vi "Begin.vi"(8 "error in":errorcluster) -> (0 "error out":errorcluster)   [LabVIEW 2020]
doc: "Called before other user functions, this VI can be used to open I/O refnums, load in file data, and do general program initialization. Notice that the <B>error out</B> terminal is simply used for data flow. Wiring it to other structures or subVIs ensures that this VI runs first."
uses:
  <vilib>/Rock Robotics/WPI/DriverStation/WPI_DriverStationRobotMode2.ctl
  <vilib>/Rock Robotics/WPI/Joystick/WPI_JoystickDeviceEnum.ctl
  Robot Global Data.vi
  <vilib>/Rock Robotics/Network Tables/NT Write String Array.vi
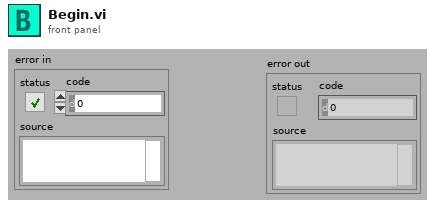
[diagram p1: front panel]
types:
  T1 = typedef "WPI_JoystickDeviceEnum.ctl" = enum16{"USB 0", "USB 1", "USB 2", "USB 3", "USB 4", "USB 5"}
  T2 = typedef "WPI_DriverStationRobotMode2.ctl" = enum16{"Autonomous Disabled", "Autonomous Enabled", "Teleop Disabled", "Teleop Enabled", "Disconnected", "Finish", "Test Disabled", "Test Enabled", "Emergency Stopped"}
  T3 = typedef "WPI_JoystickDevRef.ctl" = cluster{"Device":T1}
  T4 = typedef "numlock.ctl" = cluster{"tdms file out":refnum<k34>, "Default log level (info)":enum16{"trace", "debug", "info", "warn", "error"}}
  T5 = typedef "CTRE_PigeonIMU_DeviceRef.ctl" = cluster{"DeviceStatus":errorcluster, "Device Number":u8, "Type":T6, "Device ID":u32, "Handle":u64, "UsageFrame":u32, "Library Path":path}
  T6 = typedef "CTRE_PigeonIMU_ConnectionType.ctl" = u32
  T7 = typedef "ADIS16470 Device Reference.ctl" = cluster{"DevStatus":errorcluster, "Hardware Config":T8, "Calibration Complete":refnum<notifier>, "Status Reference":refnum<data-value>, "Position Reference":refnum<data-value>, "Velocity Reference":refnum<data-value>, "Sychronous Process VI":T12, "Cmd FIFO":refnum<k33>, "Source":T13, "Data FIFO":refnum<k33>, "Calibration Time (ms)":u32}
  T8 = typedef "ADIS16470 Hardware Configuration.ctl" = cluster{"SPI Clock Rate (Hz)":dbl, "IMU SPI Mode (3)":T9, "IMU Reset Pin":T10, "IMU SPI Bus":T11, "IMU Data Ready Pin":T10, "Stall Config":cluster{"Pow2BytesPerRead":u8, "StallTicks":u16, "CsToSclkTicks":u8}}
  T9 = typedef "WPI_SPIMode.ctl" = enum16{"Mode 0 (Clk Idle Low,Sample on Leading)", "Mode 1 (Clk Idle Low,Sample on Trailing)", "Mode 2 (Clk Idle High,Sample on Leading)", "Mode 3 (Clk Idle High,Sample on Trailing)"}
  T10 = typedef "FPGA_DIOChannel.ctl" = enum8{"DIO 0", "DIO 1", "DIO 2", "DIO 3", "DIO 4", "DIO 5", "DIO 6", "DIO 7", "DIO 8", "DIO 9", "DIO MXP 0", "DIO MXP 1", "DIO MXP 2", "DIO MXP 3", "DIO MXP 4", "DIO MXP 5", "DIO MXP 6", "DIO MXP 7", "DIO MXP 8", "DIO MXP 9", "DIO MXP 10", "DIO MXP 11", "DIO MXP 12", "DIO MXP 13", "DIO MXP 14", "DIO MXP 15", "SPI Port CS1", "SPI Port CS2", "SPI Port CS3", "SPI Port MISO", "SPI Port MOSI", "Invalid"}
  T11 = typedef "spi_bus.ctl" = enum16{"SPI On-Board, CS0", "SPI On-Board, CS1", "SPI On-Board, CS2", "SPI On-Board, CS3", "SPI MXP", "Invalid"}
  T12 = typedef "ADIS16470 Process.ctl" = refnum<vi>
  T13 = typedef "FPGA_CounterEncoderSourceConvertionLVSourceType.ctl" = cluster{"DevStatus":errorcluster, "AnalogTriggerMode?":bool, "DigitalMode":cluster{"DIO Channel":T14}, "AnalogTriggerMode":cluster{"AnalogTriggerIndex":T15, "OutputType":T16}}
  T14 = typedef "FPGA_DIODigitalSourceChannel.ctl" = enum8{"DIO 0", "DIO 1", "DIO 2", "DIO 3", "DIO 4", "DIO 5", "DIO 6", "DIO 7", "DIO 8", "DIO 9", "DIO MXP 0", "DIO MXP 1", "DIO MXP 2", "DIO MXP 3", "DIO MXP 4", "DIO MXP 5", "DIO MXP 6", "DIO MXP 7", "DIO MXP 8", "DIO MXP 9", "DIO MXP 10", "DIO MXP 11", "DIO MXP 12", "DIO MXP 13", "DIO MXP 14", "DIO MXP 15", "SPI Port CS1", "SPI Port CS2", "SPI Port CS3", "SPI Port MISO", "SPI Port MOSI", "Disabled"}
  T15 = typedef "FPGA_AnalogTriggerIndex.ctl" = enum8{"Trig 0", "Trig 1", "Trig 2", "Trig 3", "Trig 4", "Trig 5", "Trig 6", "Trig 7", "Invalid"}
  T16 = typedef "FPGA_AnalogTriggerOutType.ctl" = enum16{"InWindow", "TriggerState", "Rising", "Falling"}
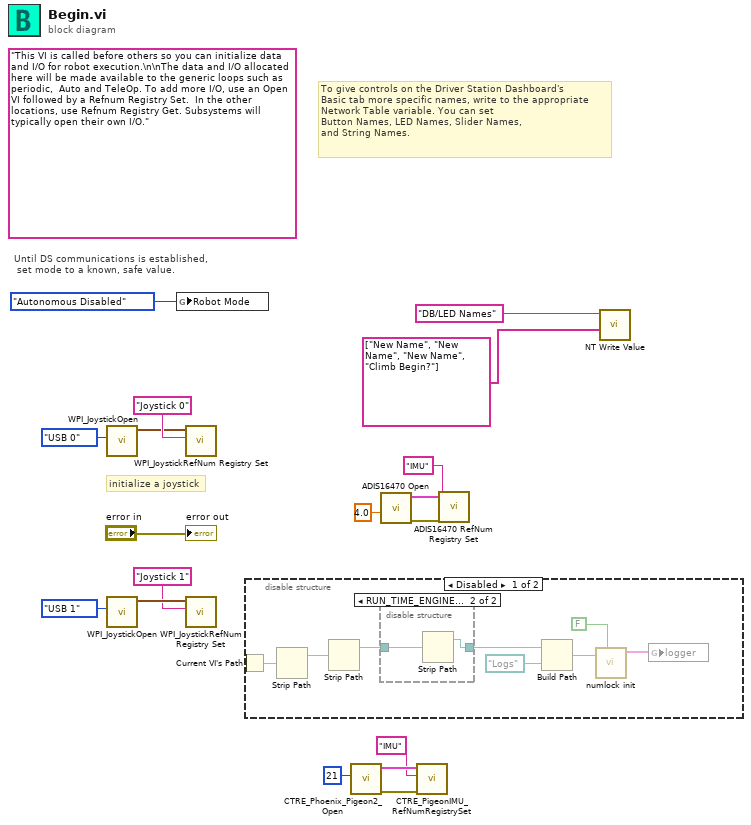
[diagram p0: block diagram]
diagram:
  (unwired) "This VI is called before others so you can initialize data and I/O for robot execution.\n\nThe data and I/O allocated here will be made available to the generic loops such as periodic,  Auto and TeleOp. To add more I/O, use an Open VI followed by a Refnum Registry Set.  In the other locations, use Refnum Registry Get. Subsystems will typically open their own I/O."
  # "To give controls on the Driver Station Dashboard's\nBasic tab more specific names, write to the appropriate\nNetwork Table variable. You can set\nButton Names, LED Names, Slider Names,\nand String Names."
  # "initialize a joystick"
  # "Until DS communications is established,\n set mode to a known, safe value."
  n1 = call <vilib>:"WPI_JoystickOpen.vi"("JoystickDevice"=WPI_JoystickDeviceEnum."USB 0") -> ("JoystickDevRef"=w16:T3)  [unwired: 10 in]
  n2 = call <vilib>:"WPI_JoystickOpen.vi"("JoystickDevice"=WPI_JoystickDeviceEnum."USB 1") -> ("JoystickDevRef"=w8:T3)  [unwired: 10 in]
  n3 = global write "Robot Global Data.vi" "Robot Mode"(WPI_DriverStationRobotMode2."Autonomous Disabled" ("Robot Mode")) -> ()
  n4 = call <vilib>:"WPI_JoystickRefNum Registry Set.vi"("refnum name"="Joystick 0", "JoystickDevRef"=w16) -> ()  [unwired: 8 in, 2 out]
  n5 = call <vilib>:"WPI_JoystickRefNum Registry Set.vi"("refnum name"="Joystick 1", "JoystickDevRef"=w8) -> ()  [unwired: 8 in, 2 out]
  n6 = disable-structure shown="Disabled" {
    frame Disabled {
      n7 = Current VI's Path() -> (path=w23:path)
      n8 = Strip Path(path=w23) -> (stripped path=w24:path)  [unwired: 1 out]
      n9 = Strip Path(path=w24) -> (stripped path=w26:path)  [unwired: 1 out]
      n10 = disable-structure shown="RUN_TIME_ENGINE==True, Default" {
        disable-tunnel: [w27 w28] -> w25
        disable-tunnel: w26 -> [w27 w29]
        frame condition #0 (active) {
        }
        frame condition #1 {
          n11 = Strip Path(path=w29) -> (stripped path=w28:path)  [unwired: 1 out]
        }
      }
      n12 = Build Path(base path=w25, name or relative path=path "Logs") -> (appended path=w21:path)
      n13 = call "numlock init.vi"("disable buffering? (T)"=FALSE, "base path"=w21) -> ("logger"=w19:T4)  [unwired: 8 in, 1 out]
      n14 = global write "Robot Global Data.vi" "logger"(w19) -> ()
    }
    frame Enabled {
    }
  }
  n15 = call <vilib>:"CTRE_Phoenix_Pigeon2_Open.vi"("Device Number"=u8 21) -> ("error out"=w2:errorcluster, "PigeonIMUDevRef"=w3:T5)  [unwired: 9 in]
  n16 = call "ADIS16470 Open.vi"("Initial Calibration Time (4s)"=4.0) -> ("error out"=w12:errorcluster, "ADIS16470DevRef"=w11:T7)  [unwired: 9 in]
  n17 = call <vilib>:"CTRE_PigeonIMU_RefNumRegistrySet.vi"("error in (no error)"=w2, "refnum name"="IMU", "PigeonIMUDevRef"=w3) -> ()  [unwired: 7 in, 2 out]
  n18 = call "ADIS16470 RefNum Registry Set.vi"("error in (no error)"=w12, "refnum name"="IMU", "ADIS16470DevRef in"=w11) -> ()  [unwired: 7 in, 2 out]
  n19 = call-poly <vilib>:"NT Write Value.vi"("String Array"=string[] ["New Name", "New Name", "New Name", "Climb Begin?"], "Name"="DB/LED Names") -> ()  [unwired: 9 in, 1 out]
  "error out" <- "error in"
